vi "Open.vi"(8 "Error In":errorcluster, 10 "SSD1306 Channels":T1, 11 "LINX Resource":T2) -> (0 "Error Out":errorcluster, 3 "LINX Resource":T2)   [LabVIEW 2014, in "LMH-LINX.lvlib" / "SSD1306.lvlib"]
doc: "Power up the SSD1306 and bring it out of reset."
uses:
  SSD1306.lvlib
  Private/Type Defs/LINX Ref.ctl
  Private/Type Defs/Platform.ctl
  Private/Type Defs/Interface.ctl
  Private/Device/Type Defs/LINX Device Config.ctl
  Private/Device/Type Defs/TCP Config.ctl
  Private/Device/Type Defs/Channels.ctl
  Private/SSD1306 Config.ctl
  Private/SSD1306 FGV State.ctl
  Peripherals/Digital/Digital Write N Chans.vi
  Peripherals/Digital/Digital Write 1 Chan.vi
  LMH-LINX.lvlib
  Private/Device/Device.lvlib
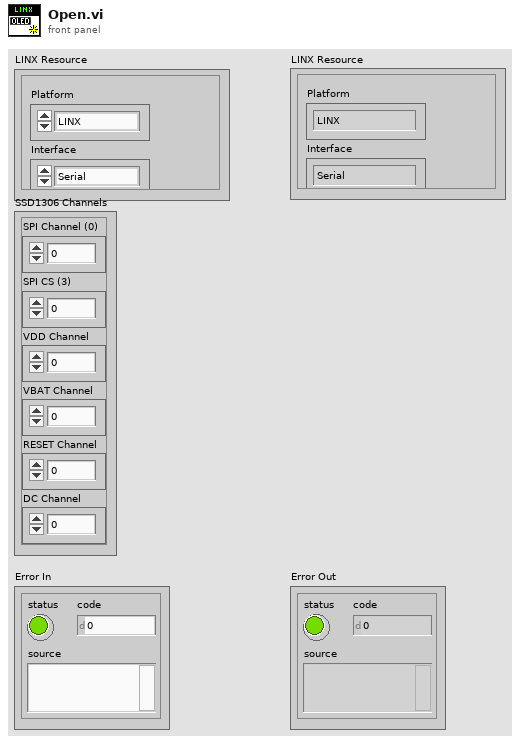
[diagram p1: front panel]
types:
  T1 = typedef "LMH-LINX.lvlib/SSD1306.lvlib/SSD1306 Config.ctl" = cluster{"SPI Channel (0)":u8, "VDD Channel":u8, "VBAT Channel":u8, "RESET Channel":u8, "DC Channel":u8, "SPI CS (3)":u8}
  T2 = typedef "LMH-LINX.lvlib/LINX Ref.ctl" = cluster{"Platform":T3, "Interface":T4, "LINX Device Config":T5}
  T3 = typedef "LMH-LINX.lvlib/Platform.ctl" = enum16{"LINX", "myRIO"}
  T4 = typedef "LMH-LINX.lvlib/Interface.ctl" = enum16{"Serial", "TCP"}
  T5 = typedef "LMH-LINX.lvlib/Device.lvlib/LINX Device Config.ctl" = cluster{"Interface":T4, "COM Port":refnum<visa-resource-name>, "TCP Configuration":T6, "Device Family":u8, "Device ID":u8, "Device Name":string, "TCP Ref":refnum<k5>, "Channels":T7}
  T6 = typedef "LMH-LINX.lvlib/Device.lvlib/TCP Config.ctl" = cluster{"IP Address":string, "Port":u16}
  T7 = typedef "LMH-LINX.lvlib/Channels.ctl" = cluster{"DI":u8[], "DO":u8[], "AI":u8[], "AO":u8[], "PWM":u8[], "QE":u8[], "UART":u8[], "I2C 2":u8[], "SPI":u8[], "CAN":u8[], "Servo":u8[], "AI Ref (V)":dbl, "AO Ref (V)":dbl, "AO Resolution (Bits)":u8}
  T8 = typedef "LMH-LINX.lvlib/SSD1306.lvlib/SSD1306 FGV State.ctl" = enum16{"Init", "Set", "Get"}
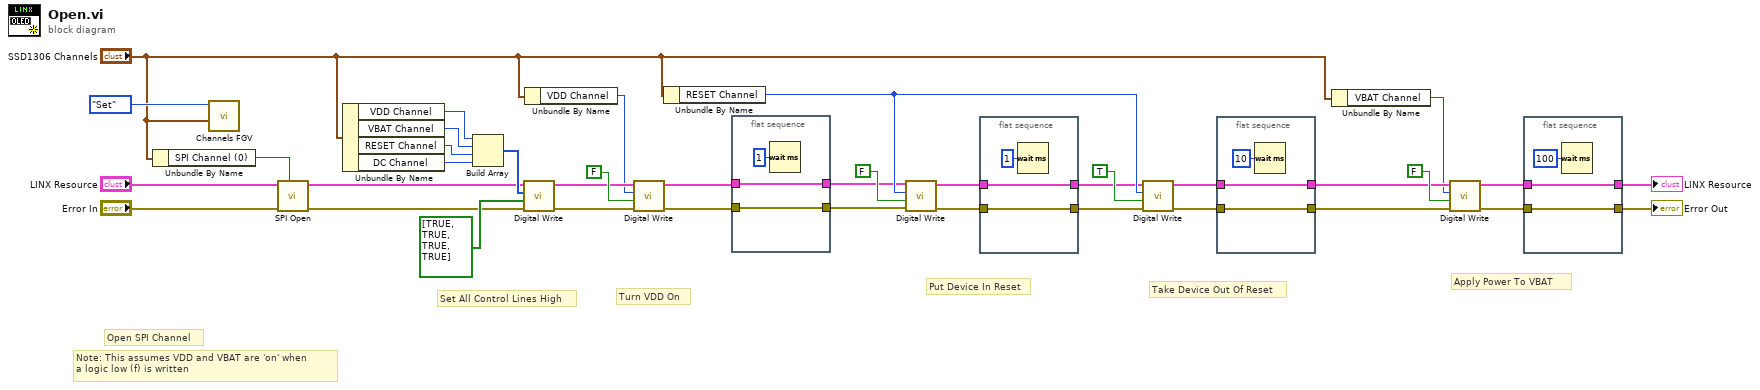
[diagram p0: block diagram]
diagram:
  # "Apply Power To VBAT"
  # "Take Device Out Of Reset"
  # "Put Device In Reset"
  # "Turn VDD On"
  # "Note: This assumes VDD and VBAT are 'on' when \na logic low (f) is written"
  # "Set All Control Lines High"
  # "Open SPI Channel"
  n1 = Unbundle By Name("SSD1306 Channels") -> ("SPI Channel (0)"=w2:u8)
  n2 = call "Channels FGV.vi"("SSD1306 Channels"="SSD1306 Channels", "SSD1306 FGV State"=SSD1306_FGV_State."Set") -> ()  [unwired: 9 in, 1 out]
  n3 = call "SPI Open.vi"("SPI Channel (0)"=w2, "Error In"="Error In", "LINX Resource"="LINX Resource") -> ("Error Out"=w4:errorcluster, "LINX Resource"=w5:T2)  [unwired: 7 in]
  n4 = Unbundle By Name("SSD1306 Channels") -> ("VDD Channel"=w31:u8, "VBAT Channel"=w37:u8, "RESET Channel"=w36:u8, "DC Channel"=w35:u8)
  n5 = Build Array(w31, w37, w36, w35) -> (w34:u8[])
  n6 = call-poly "Digital Write.vi"("Error In"=w4, "Values"=bool[] [TRUE, TRUE, TRUE, TRUE], "DO Channels"=w34, "LINX Resource"=w5) -> ("Error Out"=w32:errorcluster, "LINX Resource"=w29:T2)  [unwired: 6 in]
  n7 = Unbundle By Name("SSD1306 Channels") -> ("VDD Channel"=w27:u8)
  n8 = call-poly "Digital Write.vi"("Error In"=w32, "Output Value"=FALSE, "DO Channel"=w27, "LINX Resource"=w29) -> ("Error Out"=w9:errorcluster, "LINX Resource"=w8:T2)  [unwired: 6 in]
  n9 = Unbundle By Name("SSD1306 Channels") -> ("RESET Channel"=w21:u8)
  n10 = flat-sequence {
    tunnel: w9 -> [w40]
    tunnel: w8 -> [w39]
    tunnel: [w40] -> w7
    tunnel: [w39] -> w6
    frame #0 {
      n11 = Wait (ms)(milliseconds to wait=u32 1) -> ()  [unwired: 1 out]
    }
  }
  n12 = call-poly "Digital Write.vi"("Error In"=w7, "Output Value"=FALSE, "DO Channel"=w21, "LINX Resource"=w6) -> ("Error Out"=w26:errorcluster, "LINX Resource"=w25:T2)  [unwired: 6 in]
  n13 = flat-sequence {
    tunnel: w26 -> [w43]
    tunnel: w25 -> [w42]
    tunnel: [w43] -> w19
    tunnel: [w42] -> w20
    frame #0 {
      n14 = Wait (ms)(milliseconds to wait=u32 1) -> ()  [unwired: 1 out]
    }
  }
  n15 = call-poly "Digital Write.vi"("Error In"=w19, "Output Value"=TRUE, "DO Channel"=w21, "LINX Resource"=w20) -> ("Error Out"=w23:errorcluster, "LINX Resource"=w24:T2)  [unwired: 6 in]
  n16 = flat-sequence {
    tunnel: w23 -> [w46]
    tunnel: w24 -> [w45]
    tunnel: [w46] -> w14
    tunnel: [w45] -> w15
    frame #0 {
      n17 = Wait (ms)(milliseconds to wait=u32 10) -> ()  [unwired: 1 out]
    }
  }
  n18 = Unbundle By Name("SSD1306 Channels") -> ("VBAT Channel"=w12:u8)
  n19 = call-poly "Digital Write.vi"("Error In"=w14, "Output Value"=FALSE, "DO Channel"=w12, "LINX Resource"=w15) -> ("Error Out"=w17:errorcluster, "LINX Resource"=w16:T2)  [unwired: 6 in]
  n20 = flat-sequence {
    tunnel: w17 -> [w49]
    tunnel: w16 -> [w48]
    tunnel: [w49] -> w11
    tunnel: [w48] -> w10
    frame #0 {
      n21 = Wait (ms)(milliseconds to wait=u32 100) -> ()  [unwired: 1 out]
    }
  }
  "Error Out" <- w11
  "LINX Resource" <- w10
